vi "ReadConfigDBSubVI.vi"(0 "DB File Path":path, 1 "error in (no error)":errorcluster) -> (2 "Refnum out":T1, 3 "DB Elements":string[](array[string]), 4 "error out":errorcluster)   [LabVIEW 2016]
doc: "Reads the values of the DB section in the configuration file."
uses:
  <vilib>/Utility/config.llb/Config Data RefNum.ctl
  <vilib>/Utility/config.llb/Read Key (String).vi
  <vilib>/Utility/config.llb/NI_LVConfig.lvlib
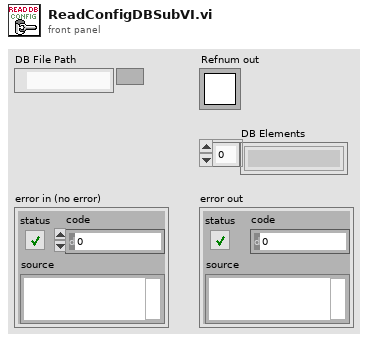
[diagram p1: front panel]
types:
  T1 = typedef "NI_LVConfig.lvlib/Config Data RefNum.ctl" = refnum<k1>
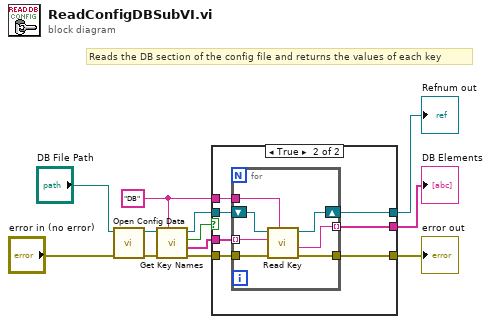
[diagram p0: block diagram]
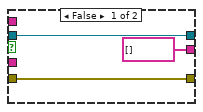
[diagram p2: hidden frame]
diagram:
  w6 = "DB" ("section")
  # "Reads the DB section of the config file and returns the values of each key"
  n1 = call <vilib>:"Open Config Data.vi"("error in (no error)"="error in (no error)", "configuration file path"="DB File Path") -> ("error out"=w8:errorcluster, "refnum"=w2:T1)  [unwired: 7 in, 1 out]
  n2 = call <vilib>:"Get Key Names.vi"("section"=w6, "error in (no error)"=w8, "refnum"=w2) -> ("error out"=w9:errorcluster, "key names"=w4:string[], "section exists?"=w3:bool, "refnum out"=w5:T1)  [unwired: 5 in]
  n3 = case shown="True" w3 {
    tunnel: w4 -> [_ w20]
    tunnel: w5 -> [w15 w22]
    tunnel: w6 -> [_ w21]
    tunnel: w9 -> [w13 w19]
    tunnel: [w13 w17] -> w10
    tunnel: [w15 w16] -> w11
    tunnel: [string[] [] w18] -> w12
    frame False {
    }
    frame True {
      n4 = for {
        tunnel: w21 -> [w28]
        tunnel: w20 -> [w27] mode=indexing
        tunnel: w19 -> [w26]
        shift-right: [w25] -> w16
        shift-left: w22 -> [w29]
        tunnel: [w24] -> w17
        tunnel: [w23] -> w18 mode=indexing
        n5 = call-poly <vilib>:"Read Key.vi"("section"=w28, "error in (no error)"=w26, "key"=w27, "refnum"=w29) -> ("error out"=w24:errorcluster, "value"=w23:string, "refnum out"=w25:T1)  [unwired: 4 in, 1 out]
      }
    }
  }
  "DB Elements" <- w12
  "Refnum out" <- w11
  "error out" <- w10
